vi "ASDEndingWavelength.vi"(0 "TCP Network Connection Refnum":refnum<k5>, 5 "Get Ending Wavelength":bool, 11 "error in (no error)":errorcluster) -> (4 "Header Code":i32, 6 "Error Code":i32, 8 "Ending Wavelength":dbl, 15 "error out":errorcluster)   [LabVIEW 2010]
panel:
  # "This is a Sub-VI of ASDTCPDemo."
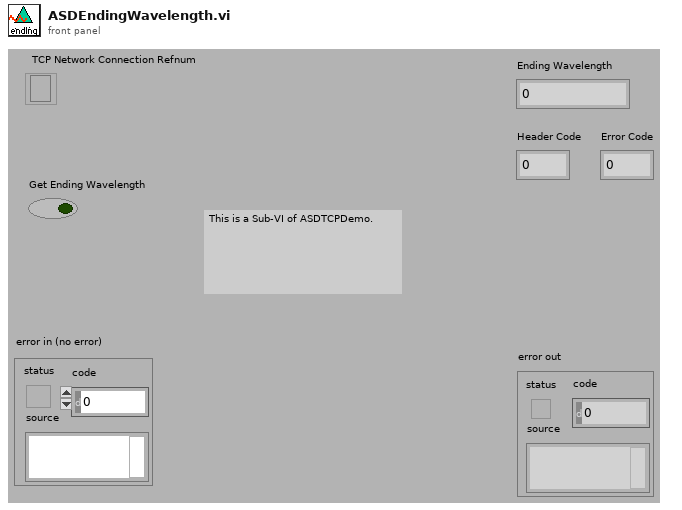
[diagram p1: front panel]
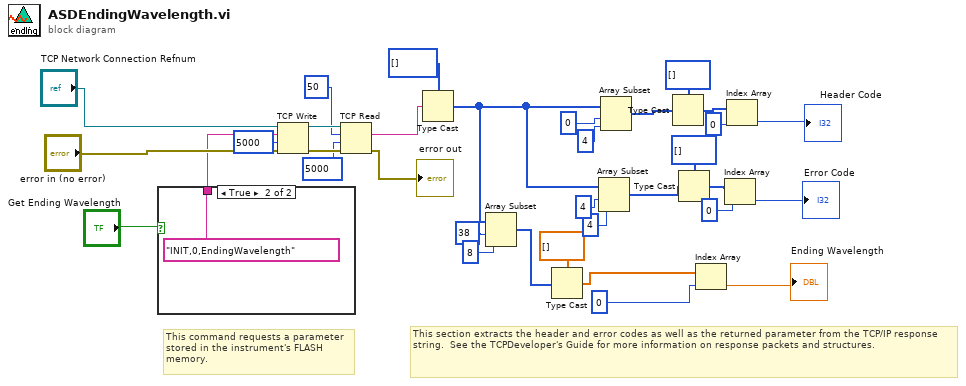
[diagram p0: block diagram]
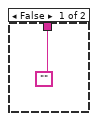
[diagram p2: hidden frame]
diagram:
  # "This section extracts the header and error codes as well as the returned parameter from the TCP/IP response string.  See the TCPDeveloper's Guide for more information on response packets and structures."
  # "This command requests a parameter stored in the instrument's FLASH memory."
  n1 = case shown="True" "Get Ending Wavelength" {
    tunnel: ["" "INIT,0,EndingWavelength"] -> w27
    frame False {
    }
    frame True {
    }
  }
  n2 = TCP Write(connection ID="TCP Network Connection Refnum", data in=w27, error in (no error)="error in (no error)", 9:5000 ("timeout ms (25000)")) -> (connection ID out=w30:refnum<k5>, error out=w31:errorcluster)  [unwired: 1 out]
  n3 = TCP Read(connection ID=w30, bytes to read=50, error in (no error)=w31, 9:5000 ("timeout ms (25000)")) -> (data out=w29:string, error out=→"error out":errorcluster)  [unwired: 1 in, 1 out]
  n4 = Type Cast(type=u8[] [], x=w29) -> (*(type *) &x=w15:u8[])
  n5 = Array Subset(array=w15, index=38, length=8 ("index")) -> (w11:u8[])
  n6 = Type Cast(type=dbl[] [], x=w11) -> (*(type *) &x=w19:dbl[])
  n7 = Array Subset(array=w15, index=4, length=4 ("index")) -> (w4:u8[])
  n8 = Array Subset(array=w15, index=0 ("start index (0)"), length=4) -> (w10:u8[])
  n9 = Type Cast(type=i32[] [], x=w10) -> (*(type *) &x=w9:i32[])
  n10 = Type Cast(type=i32[] [], x=w4) -> (*(type *) &x=w5:i32[])
  n11 = Index Array(array=w19, index=0) -> (element=→"Ending Wavelength":dbl)
  n12 = Index Array(array=w5, index=0) -> (element=→"Error Code":i32)
  n13 = Index Array(array=w9, index=0) -> (element=→"Header Code":i32)
